vi "Update Clock Main.vi"(8 "error in (no error)":errorcluster, 9 "Reinit":bool, 10 "Timestamp Pair":T1, 11 "CIFCorePlugin in":refnum<class "CIFCorePlugin.lvclass">) -> (0 "error out":errorcluster, 3 "CIFCorePlugin out":refnum<class "CIFCorePlugin.lvclass">)   [LabVIEW 2021, in "CIFCorePlugin.lvclass"]
doc: "It registers an update of a time pair to track an external clock. \n \nThe ClockID can be read from the system and is set via gRPC for the plugin.\nSystem Time is the OS time. External time is the clock to be tracked. \nIf this is the first update or if external time has jumped (had a discontinuity, gone backwards, etc) then the reinit should be set true.\n\nUpdates will be passed to the CIF manager on the system. Then the clock conversion will be updated and automatically passed to all plugins. \n\nThis VI must be called from the main loop. It will pass the time pair to the gRPC monitoring loop which will update the manager."
uses:
  CIFCorePlugin.lvclass
  CIFCorePlugin.lvclass/CIFCorePlugin.ctl
  <vilib>/CIF Foundation/CIF Utilities/Time/Typedef/Timestamp Pair.ctl
  <vilib>/CIF Foundation/CIF Utilities/Time/Time_CIF_U.lvlib
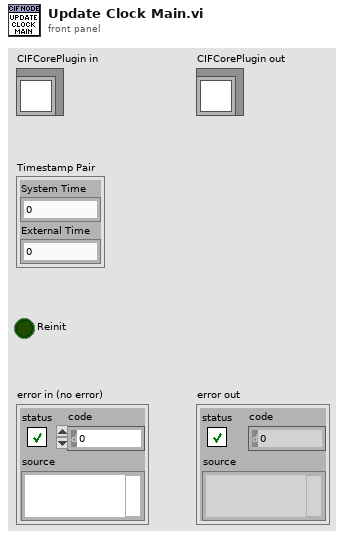
[diagram p1: front panel]
types:
  T1 = typedef "Time_CIF_U.lvlib/Timestamp Pair.ctl" = cluster{"System Time":i64, "External Time":i64}
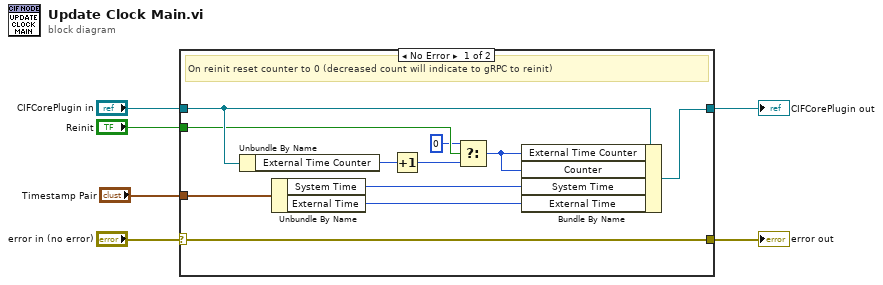
[diagram p0: block diagram]
diagram:
  n1 = case shown="No Error" "error in (no error)" {
    selector: "error in (no error)" -> [w17 w19]
    tunnel: [w17 w19] -> w5
    tunnel: [w14 w18] -> w3
    tunnel: "CIFCorePlugin in" -> [w15 w18]
    tunnel: "Reinit" -> [w11 _]
    tunnel: "Timestamp Pair" -> [w9 _]
    frame No Error {
      # "On reinit reset counter to 0 (decreased count will indicate to gRPC to reinit)"
      n2 = Unbundle By Name(w15) -> ("External Time Counter"=w16:u64)
      n3 = Unbundle By Name(w9) -> ("System Time"=w8:i64, "External Time"=w7:i64)
      n4 = Increment(x=w16) -> (x+1=w13:u64)
      n5 = Select(t=u64 0, s=w11, f=w13) -> (s? t:f=w12:u64)
      n6 = Bundle By Name(cluster=w15, "External Time Counter"=w12, "Counter"=w12, "System Time"=w8, "External Time"=w7) -> (w14:refnum<class "CIFCorePlugin.lvclass">)
    }
    frame Error {
    }
  }
  "error out" <- w5
  "CIFCorePlugin out" <- w3
